vi "Plot_Server_Data.vi"() -> ()   [LabVIEW 2021]
uses:
  Anemometry/Anemometry Sub Vis/Controls/Server_Comms.ctl
  Anemometry/Anemometry Sub Vis/File/Setup_Filetype.ctl
  Anemometry/Anemometry Sub Vis/Globals/Preference_global.vi
  ADAM Server/ADAM_Global.vi
panel:
  out "LastUpdated":string="Tue, May 12, 2015 at 11:28"
  in  "Throwback\n(mins)":dbl format="%.1f"
  in  "stop":bool=TRUE
  in  "Mode":T1(ring)=enum."Display data over specified period:"
  in  "History\n(mins)":dbl=20.0 format="%.1f"
  in  "Save plot number":T2(ring)
  out "Plot 3 Chs":string[](array[string])
  out "Plot 2 Chs":string[](array[string])
  out "Plot 1 Chs":string[](array[string])
  in  "Selector 1":i32[](listbox)
  in  "Search 1":string caption="Search:"
  in  "Search 2":string caption="Search:"
  in  "Search 3":string caption="Search:"
  in  "Selector 3":i32[](listbox)
  in  "Selector 2":i32[](listbox)
  in  "Precision":i32=2
  in  "Save 3":bool
  in  "palette3":i32(ring)=5 caption="Palette" items=["Strong", "Dark", "Light", "Pastel", "Pale", "Brash", "Clean", "Tidy"]
  out "Plot 3":cluster{"Times":dbl[], "Output array":dbl[]}[](graph)
  in  "Save 2":bool
  in  "palette2":i32(ring)=5 caption="Palette" items=["Strong", "Dark", "Light", "Pastel", "Pale", "Brash", "Clean", "Tidy"]
  out "Plot 2":cluster{"Times":dbl[], "Output array":dbl[]}[](graph)
  in  "Save 1":bool
  in  "palette1":i32(ring)=5 caption="Palette" items=["Strong", "Dark", "Light", "Pastel", "Pale", "Brash", "Clean", "Tidy"]
  out "Plot 1":cluster{"Times":dbl[], "Output array":dbl[]}[](graph)
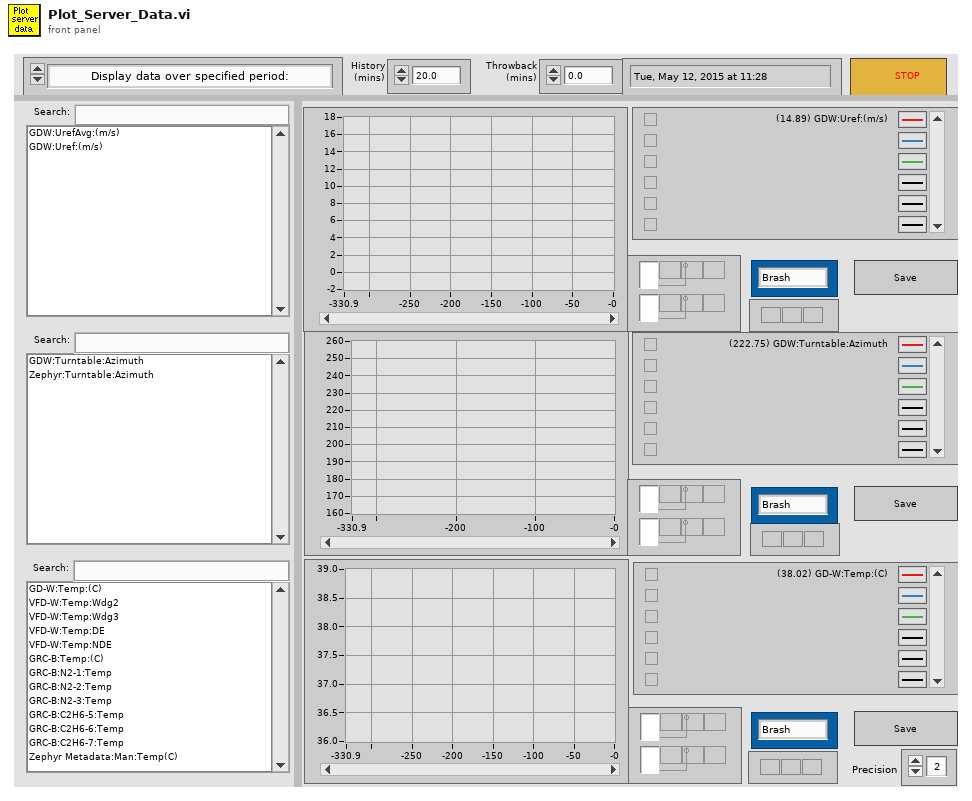
[diagram p1: front panel]
types:
  T1 = enum16{"Display full time history", "Display data over specified period:"}
  T2 = enum16{"Save Plot 1", "Save Plot 2", "Save Plot 3"}
  T3 = typedef "Server_Comms.ctl" = enum16{"Do Not Link To Server", "Server Link Healthy"}
  T4 = typedef "Setup_Filetype.ctl" = enum16{"Measurement Setups", "Calibration Setups", "General", "Results File Plotter Setups", "Speed Calib Tweaks"}
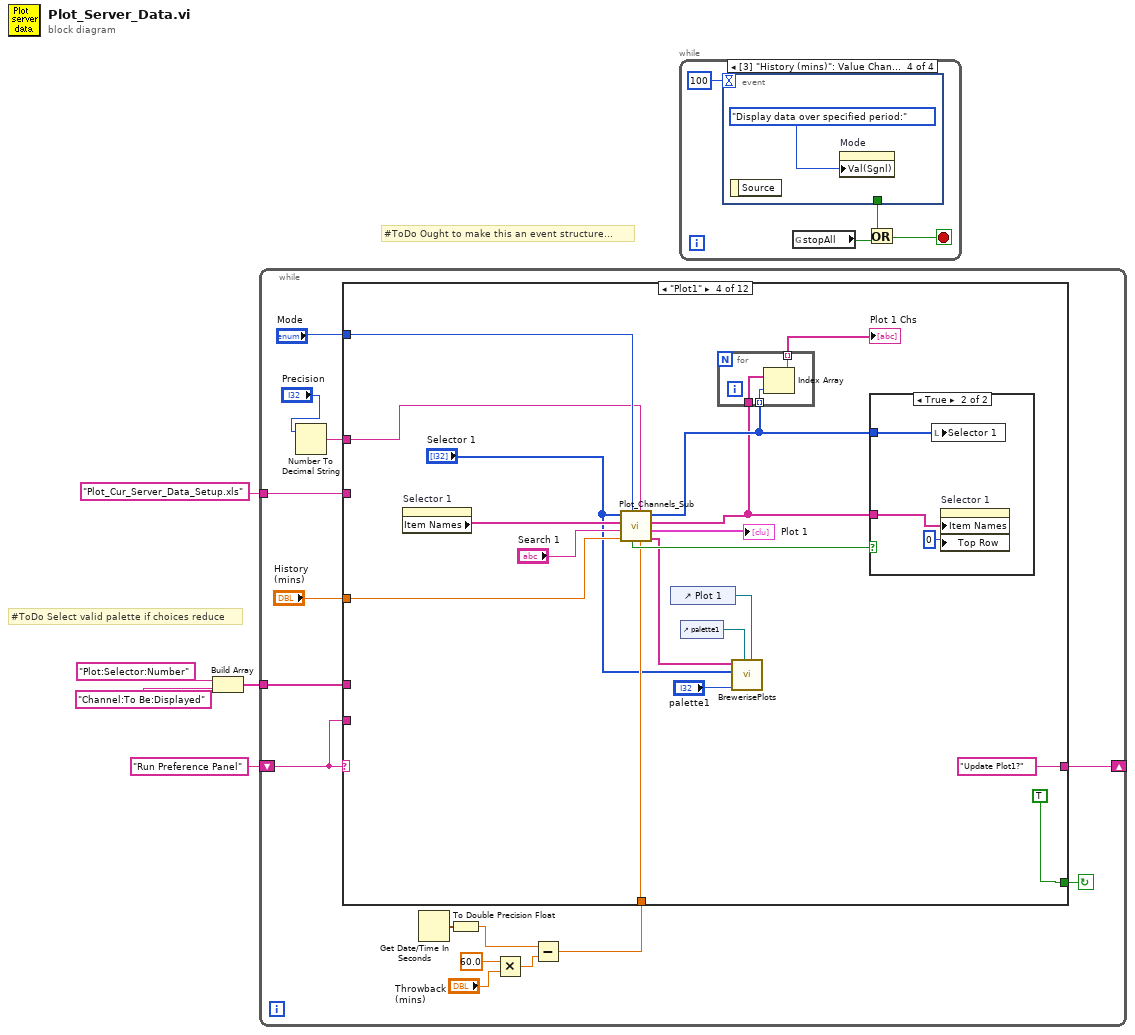
[diagram p0: block diagram]
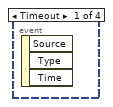
[diagram p2: hidden frame]
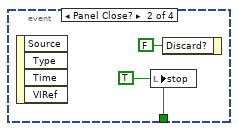
[diagram p3: hidden frame]
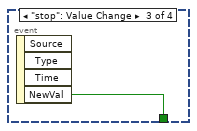
[diagram p4: hidden frame]
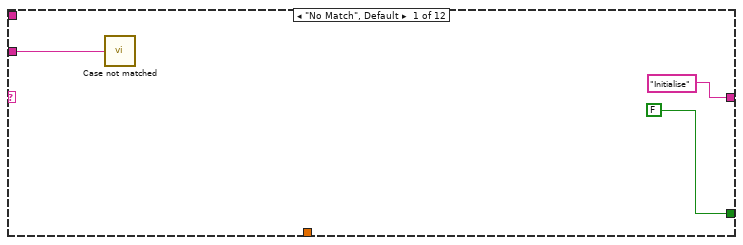
[diagram p5: hidden frame]
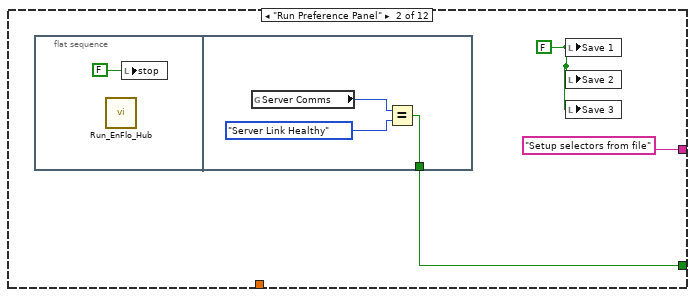
[diagram p6: hidden frame]
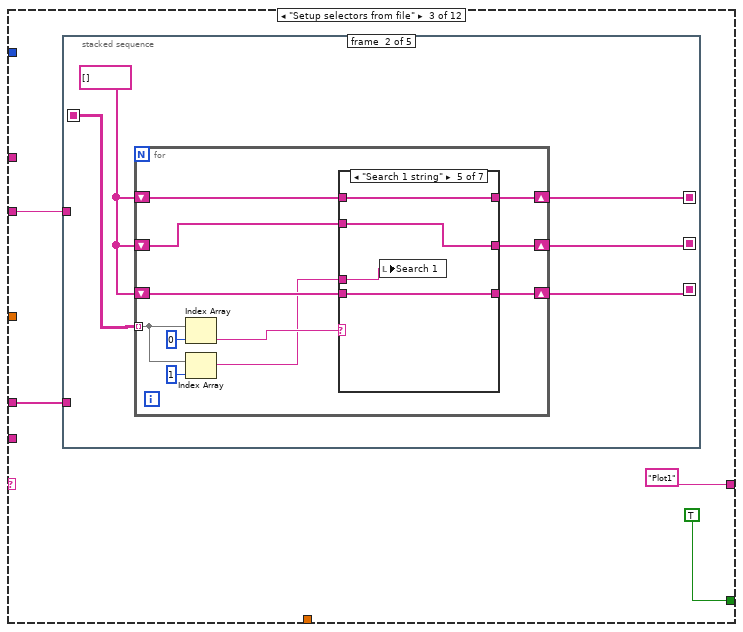
[diagram p7: hidden frame]
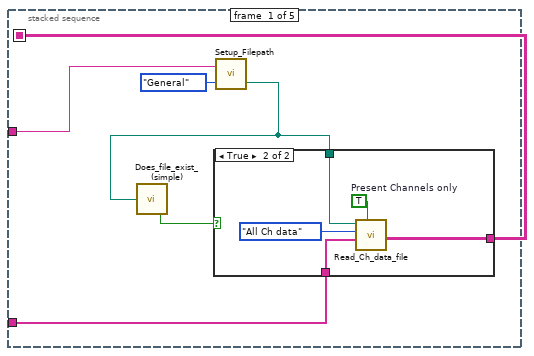
[diagram p8: hidden frame]
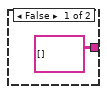
[diagram p9: hidden frame]
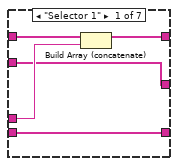
[diagram p10: hidden frame]
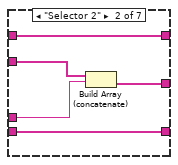
[diagram p11: hidden frame]
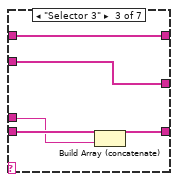
[diagram p12: hidden frame]
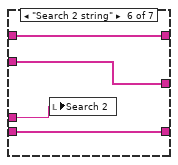
[diagram p14: hidden frame]
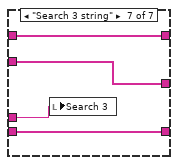
[diagram p15: hidden frame]
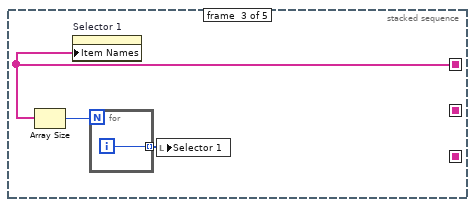
[diagram p16: hidden frame]
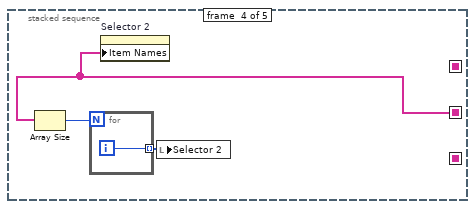
[diagram p17: hidden frame]
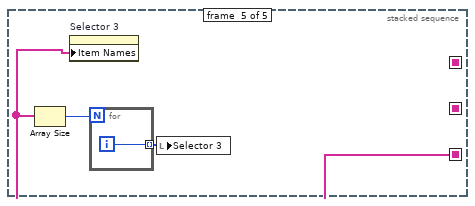
[diagram p18: hidden frame]
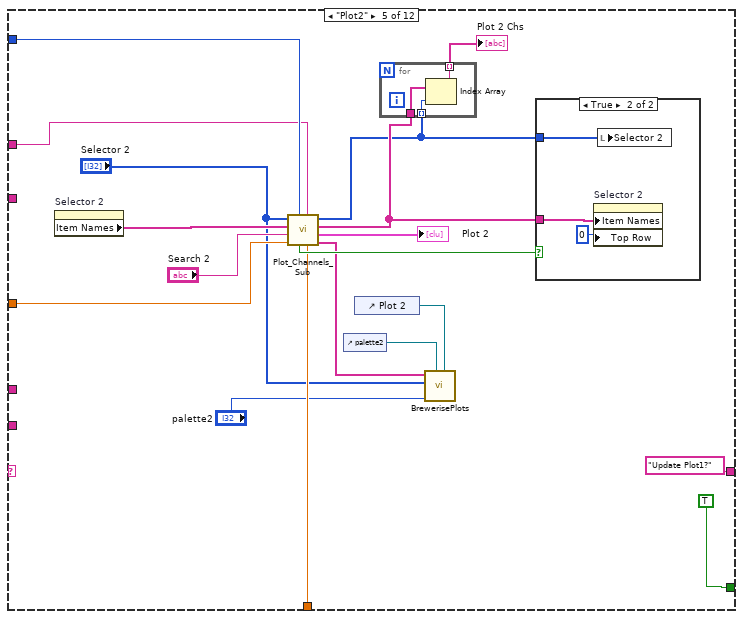
[diagram p20: hidden frame]
diagram:
  # "#ToDo Select valid palette if choices reduce"
  # "#ToDo Ought to make this an event structure..."
  n1 = Build Array("Plot:Selector:Number", "Channel:To Be:Displayed") -> (w2:string[])
  n2 = while {
    shift-left: "Run Preference Panel" -> [w18]
    shift-right: [w19] -> _
    tunnel: w2 -> [w15]
    tunnel: "Plot_Cur_Server_Data_Setup.xls" -> [w14]
    stop <- w20 continue-if-true
    n3 = Number To Decimal String(number="Precision") -> (decimal integer string=w12:string)  [unwired: 1 out]
    n4 = Get Date/Time In Seconds() -> (seconds since 1Jan1904=w11:timestamp)
    n5 = To Double Precision Float(number=w11) -> (double precision float=w7:dbl)
    n6 = Multiply(x=60.0, y="Throwback\n(mins)") -> (x*y=w8:dbl)
    n7 = Subtract(x=w7, y=w8) -> (x-y=w6:dbl)
    n8 = case shown="\"Plot1\"" w18 {
      tunnel: [FALSE w25 TRUE TRUE TRUE TRUE TRUE TRUE TRUE TRUE w319 w385] -> w20
      tunnel: ["Initialise" "Setup selectors from file" "Plot1" "Update Plot1?" "Update Plot1?" "Update Plot1?" w181 w207 w232 w267 w320 "Update Plot1?" ("t")] -> w19
      tunnel: w18 -> [w21 _ _ _ _ _ _ _ _ _ _ _]
      tunnel: "Mode" -> [_ _ _ w116 w143 w167 _ _ _ _ _ _]
      tunnel: "History\n(mins)" -> [_ _ _ w115 w142 w166 _ _ _ _ _ _]
      tunnel: w15 -> [_ _ w31 _ _ _ _ _ _ _ _ w389]
      tunnel: w14 -> [_ _ w32 _ _ _ _ _ _ _ _ w388]
      tunnel: w12 -> [_ _ _ w111 w135 w159 _ _ _ _ _ _]
      tunnel: w6 -> [_ _ _ w110 w134 w158 _ _ _ _ _ _]
      frame "No Match", Default {
        n9 = call "Case not matched.vi"("Case Name not Matched"=w21) -> ()
      }
      frame "Run Preference Panel" {
        w24 = FALSE ("Save 1")
        n10 = flat-sequence {
          tunnel: [w28] -> w25
          frame #0 {
            n11 = call "Run_EnFlo_Hub.vi"() -> ()  [unwired: 1 in, 7 out]
            n12 = local write "stop"(FALSE ("stop")) -> ()
          }
          frame #1 {
            n13 = global read "Preference_global.vi" "Server Comms"() -> (w29:T3)
            n14 = Equal?(x=w29, y=Server_Comms."Server Link Healthy" ("Server Comms")) -> (x = y?=w28:bool)
          }
        }
        n15 = local write "Save 1"(w24) -> ()
        n16 = local write "Save 2"(w24) -> ()
        n17 = local write "Save 3"(w24) -> ()
      }
      frame "Setup selectors from file" {
        n18 = stacked-sequence {
          seq-local: [w38 _ _ _ _] -> [_ w51 _ _ _]
          seq-local: [_ w49 _ _ _] -> [_ _ w95 _ _]
          seq-local: [_ w47 _ _ _] -> [_ _ _ w97 _]
          seq-local: [_ w48 _ _ _] -> [_ _ _ _ w101]
          tunnel: w32 -> [w37 _ _ _ _]
          tunnel: w31 -> [w39 _ _ _ _]
          frame #0 {
            n19 = call "Setup_Filepath.vi"("Setup File Type"=Setup_Filetype."General", "Filename in"=w37) -> ("Filename Out"=w36:path)  [unwired: 1 out]
            n20 = call "Does_file_exist_(simple).vi"("Pathname"=w36) -> ("exists?"=w40:bool)
            n21 = case shown="True" w40 {
              tunnel: w36 -> [_ w46]
              tunnel: w39 -> [_ w45]
              tunnel: [string[][] [] ("Channel Values") w42] -> w38
              frame False {
              }
              frame True {
                w44 = TRUE  # Present Channels only
                n22 = call "Read_Ch_data_file.vi"("Present Channels only"=w44, "Present Channels"=w45, "Output"=enum16{"All Ch data", "The last few rows"}."All Ch data", "Filename"=w46) -> ("Channel Values"=w42:string[][])  [unwired: 1 in, 4 out]
              }
            }
          }
          frame #1 {
            w50 = string[] []
            n23 = for {
              shift-right: [w57] -> w49
              shift-left: w50 -> [w58]
              tunnel: w51 -> [w59] mode=indexing
              shift-right: [w55] -> w47
              shift-left: w50 -> [w56]
              shift-right: [w53] -> w48
              shift-left: w50 -> [w54]
              n24 = Index Array(array=w59, index=0 ("Index")) -> (element=w61:string)
              n25 = Index Array(array=w59, index=1 ("Index")) -> (element=w52:string)
              n26 = case shown="\"Search 1 string\"" w61 {
                tunnel: w58 -> [w67 w72 w73 w79 w83 w87 w91]
                tunnel: [w66 w72 w73 w79 w83 w87 w91] -> w57
                tunnel: w52 -> [w65 w69 w75 _ w81 w85 w89]
                tunnel: w56 -> [w64 w70 w74 w80 w84 w88 w92]
                tunnel: [w64 w68 w74 w80 w84 w88 w92] -> w55
                tunnel: w54 -> [w63 w71 w77 w78 w82 w86 w90]
                tunnel: [w63 w71 w76 w78 w82 w86 w90] -> w53
                frame "Selector 1" {
                  n27 = Build Array (concatenate)(w67, w65) -> (w66:string[])
                }
                frame "Selector 2" {
                  n28 = Build Array (concatenate)(w70, w69) -> (w68:string[])
                }
                frame "Selector 3" {
                  n29 = Build Array (concatenate)(w77, w75) -> (w76:string[])
                }
                frame "No Match", Default {
                }
                frame "Search 1 string" {
                  n30 = local write "Search 1"(w81) -> ()
                }
                frame "Search 2 string" {
                  n31 = local write "Search 2"(w85) -> ()
                }
                frame "Search 3 string" {
                  n32 = local write "Search 3"(w89) -> ()
                }
              }
            }
          }
          frame #2 {
            n33 = Array Size(array=w95) -> (size(s)=w94:i32)
            n34 = property on="Selector 1" class="LstBox (strict)"("Item Names"=w95) -> ()  [unwired: 2 in, 2 out]
            n35 = for {
              N: w94 -> [_]
              tunnel: [w96] -> w93 mode=indexing
              i -> [w96]
            }
            n36 = local write "Selector 1"(w93) -> ()
          }
          frame #3 {
            n37 = Array Size(array=w97) -> (size(s)=w99:i32)
            n38 = for {
              N: w99 -> [_]
              tunnel: [w100] -> w98 mode=indexing
              i -> [w100]
            }
            n39 = property on="Selector 2" class="LstBox (strict)"("Item Names"=w97) -> ()  [unwired: 2 in, 2 out]
            n40 = local write "Selector 2"(w98) -> ()
          }
          frame #4 {
            n41 = Array Size(array=w101) -> (size(s)=w103:i32)
            n42 = property on="Selector 3" class="LstBox (strict)"("Item Names"=w101) -> ()  [unwired: 2 in, 2 out]
            n43 = for {
              N: w103 -> [_]
              tunnel: [w104] -> w102 mode=indexing
              i -> [w104]
            }
            n44 = local write "Selector 3"(w102) -> ()
          }
        }
      }
      frame "Plot1" {
        n45 = property on="Selector 1" class="LstBox (strict)"() -> ("Item Names"=w117:string[])  [unwired: 2 in, 2 out]
        n46 = call "Plot_Channels_Sub.vi"("End Time"=w110, "precision"=w111, "Mode"=w116, "History (min)"=w115, "Search String"="Search 1", "Selector List In"=w117, "Selector array In"="Selector 1") -> ("Plot Legend"=w107:string[], "Plot"=→"Plot 1":cluster{"Times":dbl[], "Output array":dbl[]}[], "Selector List Out"=w113:string[], "Selector array Out"=w114:i32[], "Selector Changed?"=w119:bool)
        n47 = control-ref of="Plot 1"() -> (w109:refnum<vi>)
        n48 = control-ref of="palette1"() -> (w108:refnum<vi>)
        n49 = for {
          tunnel: w114 -> [w125] mode=indexing
          tunnel: w113 -> [w124]
          tunnel: [w123] -> w112 mode=indexing
          n50 = Index Array(array=w124, index=w125) -> (element=w123:string)
        }
        "Plot 1 Chs" <- w112
        n51 = call "BrewerisePlots.vi"("graphRefnum"=w109, "paletteRefnum"=w108, "paletteNum"="palette1", "Series"="Selector 1", "Plot Legends"=w107) -> ()  [unwired: 7 in]
        n52 = case shown="True" w119 {
          tunnel: w113 -> [_ w128]
          tunnel: w114 -> [_ w127]
          frame False {
          }
          frame True {
            n53 = local write "Selector 1"(w127) -> ()
            n54 = property on="Selector 1" class="LstBox (strict)"("Item Names"=w128, "Top Row"=0) -> ()  [unwired: 2 in, 2 out]
          }
        }
      }
      frame "Plot2" {
        n55 = property on="Selector 2" class="LstBox (strict)"() -> ("Item Names"=w139:string[])  [unwired: 2 in, 2 out]
        n56 = call "Plot_Channels_Sub.vi"("End Time"=w134, "precision"=w135, "Mode"=w143, "History (min)"=w142, "Search String"="Search 2", "Selector List In"=w139, "Selector array In"="Selector 2") -> ("Plot Legend"=w131:string[], "Plot"=→"Plot 2":cluster{"Times":dbl[], "Output array":dbl[]}[], "Selector List Out"=w138:string[], "Selector array Out"=w137:i32[], "Selector Changed?"=w144:bool)
        n57 = control-ref of="palette2"() -> (w132:refnum<vi>)
        n58 = control-ref of="Plot 2"() -> (w133:refnum<vi>)
        n59 = for {
          tunnel: w137 -> [w149] mode=indexing
          tunnel: w138 -> [w148]
          tunnel: [w147] -> w136 mode=indexing
          n60 = Index Array(array=w148, index=w149) -> (element=w147:string)
        }
        "Plot 2 Chs" <- w136
        n61 = call "BrewerisePlots.vi"("graphRefnum"=w133, "paletteRefnum"=w132, "paletteNum"="palette2", "Series"="Selector 2", "Plot Legends"=w131) -> ()  [unwired: 7 in]
        n62 = case shown="True" w144 {
          tunnel: w138 -> [_ w151]
          tunnel: w137 -> [_ w152]
          frame False {
          }
          frame True {
            n63 = property on="Selector 2" class="LstBox (strict)"("Item Names"=w151, "Top Row"=0) -> ()  [unwired: 2 in, 2 out]
            n64 = local write "Selector 2"(w152) -> ()
          }
        }
      }
      frame "Plot3" {
        n65 = property on="Selector 3" class="LstBox (strict)"() -> ("Item Names"=w163:string[])  [unwired: 2 in, 2 out]
        n66 = call "Plot_Channels_Sub.vi"("End Time"=w158, "precision"=w159, "Mode"=w167, "History (min)"=w166, "Search String"="Search 3", "Selector List In"=w163, "Selector array In"="Selector 3") -> ("Plot Legend"=w155:string[], "Plot"=→"Plot 3":cluster{"Times":dbl[], "Output array":dbl[]}[], "Selector List Out"=w162:string[], "Selector array Out"=w161:i32[], "Selector Changed?"=w168:bool)
        n67 = control-ref of="Plot 3"() -> (w157:refnum<vi>)
        n68 = control-ref of="palette3"() -> (w156:refnum<vi>)
        n69 = for {
          tunnel: w161 -> [w173] mode=indexing
          tunnel: w162 -> [w172]
          tunnel: [w171] -> w160 mode=indexing
          n70 = Index Array(array=w172, index=w173) -> (element=w171:string)
        }
        "Plot 3 Chs" <- w160
        n71 = call "BrewerisePlots.vi"("graphRefnum"=w157, "paletteRefnum"=w156, "paletteNum"="palette3", "Series"="Selector 3", "Plot Legends"=w155) -> ()  [unwired: 7 in]
        n72 = case shown="True" w168 {
          tunnel: w162 -> [_ w175]
          tunnel: w161 -> [_ w176]
          frame False {
          }
          frame True {
            n73 = local write "Selector 3"(w176) -> ()
            n74 = property on="Selector 3" class="LstBox (strict)"("Item Names"=w175, "Top Row"=0) -> ()  [unwired: 2 in, 2 out]
          }
        }
      }
      frame "Update Plot1?" {
        n75 = while {
          shift-right: [w201] -> w188
          shift-left: _ -> [w198]
          shift-right: [w200] -> w190
          shift-left: _ -> [w199]
          tunnel: [w199] -> w189
          tunnel: [w198] -> w187
          shift-right: [w196] -> w178
          shift-left: _ -> [w195]
          tunnel: [w195] -> w179
          stop <- FALSE continue-if-true
          n76 = local read "Selector 1"() -> (w201:i32[])
          n77 = local read "palette1"() -> (w196:i32)
          n78 = local read "Search 1"() -> (w200:string)
        }
        n79 = case shown="False" "Save 1" {
          tunnel: ["Update Plot2?" "Save Plot" ("t")] -> w180
          frame False {
          }
          frame True {
            n80 = local write "Save plot number"(T2."Save Plot 1" ("Save plot number")) -> ()
          }
        }
        n81 = Equal?(x=w178, y=w179) -> (x = y?=w177:bool)
        n82 = Equal?(x=w188, y=w187) -> (x = y?=w185:bool)
        n83 = Equal?(x=w189, y=w190) -> (x = y?=w186:bool)
        n84 = Compound Arithmetic op=AND(w177, w185, w186) -> (w184:bool)
        n85 = Select(t=w180, s=w184, f="Plot1") -> (s? t:f=w181:string)
      }
      frame "Update Plot2?" {
        n86 = while {
          shift-right: [w226] -> w213
          shift-left: _ -> [w223]
          shift-right: [w225] -> w215
          shift-left: _ -> [w224]
          tunnel: [w224] -> w214
          tunnel: [w223] -> w212
          shift-right: [w221] -> w203
          shift-left: _ -> [w220]
          tunnel: [w220] -> w204
          stop <- FALSE continue-if-true
          n87 = local read "Selector 2"() -> (w226:i32[])
          n88 = local read "Search 2"() -> (w225:string)
          n89 = local read "palette2"() -> (w221:i32)
        }
        n90 = case shown="False" "Save 2" {
          tunnel: ["Update Plot3?" "Save Plot" ("t")] -> w205
          frame False {
          }
          frame True {
            n91 = local write "Save plot number"(T2."Save Plot 2" ("Save plot number")) -> ()
          }
        }
        n92 = Equal?(x=w203, y=w204) -> (x = y?=w202:bool)
        n93 = Equal?(x=w213, y=w212) -> (x = y?=w210:bool)
        n94 = Equal?(x=w214, y=w215) -> (x = y?=w211:bool)
        n95 = Compound Arithmetic op=AND(w202, w210, w211) -> (w209:bool)
        n96 = Select(t=w205, s=w209, f="Plot2") -> (s? t:f=w207:string)
      }
      frame "Update Plot3?" {
        n97 = while {
          shift-right: [w251] -> w238
          shift-left: _ -> [w248]
          shift-right: [w250] -> w240
          shift-left: _ -> [w249]
          tunnel: [w249] -> w239
          tunnel: [w248] -> w237
          shift-right: [w246] -> w229
          shift-left: _ -> [w245]
          tunnel: [w245] -> w228
          stop <- FALSE continue-if-true
          n98 = local read "Selector 3"() -> (w251:i32[])
          n99 = local read "Search 3"() -> (w250:string)
          n100 = local read "palette3"() -> (w246:i32)
        }
        n101 = case shown="False" "Save 3" {
          tunnel: ["What to do next?" "Save Plot" ("t")] -> w230
          frame False {
          }
          frame True {
            n102 = local write "Save plot number"(T2."Save Plot 3" ("Save plot number")) -> ()
          }
        }
        n103 = Equal?(x=w238, y=w237) -> (x = y?=w235:bool)
        n104 = Equal?(x=w239, y=w240) -> (x = y?=w236:bool)
        n105 = Equal?(x=w229, y=w228) -> (x = y?=w227:bool)
        n106 = Compound Arithmetic op=AND(w227, w235, w236) -> (w234:bool)
        n107 = Select(t=w230, s=w234, f="Plot3") -> (s? t:f=w232:string)
      }
      frame "What to do next?" {
        n108 = Wait (ms)(milliseconds to wait=u32 300) -> ()  [unwired: 1 out]
        n109 = while {
          shift-right: [w283] -> _
          shift-left: _ -> [w282]
          shift-right: [w281] -> _
          shift-left: _ -> [w280]
          shift-right: [w273] -> _
          shift-left: _ -> [w272]
          tunnel: [w275] -> w266
          shift-right: [w269] -> w256
          shift-left: _ -> [w270]
          stop <- FALSE continue-if-true
          n110 = local read "History\n(mins)"() -> (w283:dbl)
          n111 = local read "Mode"() -> (w281:T1)
          n112 = Equal?(x=w283, y=w282) -> (x = y?=w279:bool)
          n113 = Equal?(x=w280, y=w281) -> (x = y?=w278:bool)
          n114 = And(x=w279, y=w278) -> (x .and. y?=w277:bool)
          n115 = Select(t=w272, s=w277, f=0) -> (s? t:f=w274:i32)
          n116 = case shown="5" w274 {
            tunnel: ["Plot1" "Plot2" "Plot3" "Update Plot1?" "Update Plot1?" "Update Plot1?" "Update Plot1?"] -> w275
            tunnel: w274 -> [w286 w290 w294 w300 w306 w312 _]
            tunnel: [w285 w289 w293 w299 w305 w311 0] -> w273
            tunnel: w270 -> [w284 w288 w292 w297 w303 w308 w315]
            tunnel: [w284 w288 w292 w296 w302 w309 w314] -> w269
            frame 0, Default {
              n117 = Increment(x=w286) -> (x+1=w285:i32)
            }
            frame 1 {
              n118 = Increment(x=w290) -> (x+1=w289:i32)
            }
            frame 2 {
              n119 = Increment(x=w294) -> (x+1=w293:i32)
            }
            frame 3 {
              n120 = Add(x=w297, y=1) -> (x+y=w296:i32)
              n121 = Increment(x=w300) -> (x+1=w299:i32)
            }
            frame 4 {
              n122 = Add(x=w303, y=1) -> (x+y=w302:i32)
              n123 = Increment(x=w306) -> (x+1=w305:i32)
            }
            frame 5 {
              n124 = Add(x=w308, y=1) -> (x+y=w309:i32)
              n125 = Increment(x=w312) -> (x+1=w311:i32)
            }
            frame 6 {
              n126 = Add(x=w315, y=1) -> (x+y=w314:i32)
            }
          }
        }
        n127 = Get Date/Time String(date format (0)=enum16{"short", "long", "abbreviated"}."abbreviated") -> (date string=w263:string, time string=w264:string)  [unwired: 2 out]
        n128 = Concatenate Strings(w263, " at " ("Substring"), w264) -> (→"LastUpdated":string)
        n129 = Quotient & Remainder(x=w256, y=500) -> (x-y*floor(x/y)=w260:i32)  [unwired: 1 out]
        n130 = global read "ADAM_Global.vi" "stopAll"() -> (w252:bool)
        n131 = Equal To 0?(x=w260) -> (x = 0?=w258:bool)
        n132 = Compound Arithmetic op=OR("stop", w258, w252) -> (w257:bool)
        n133 = Select(t="Save Channel Names", s=w257, f=w266) -> (s? t:f=w267:string)
      }
      frame "Save Plot" {
        n134 = stacked-sequence {
          seq-local: [w331 _] -> [_ w359]
          seq-local: [w326 _] -> [_ w361]
          seq-local: [w330 _] -> [_ w360]
          seq-local: [w321 _] -> [_ w349]
          tunnel: ["What to do next?" _] -> w320
          tunnel: [TRUE _] -> w319
          frame #0 {
            n135 = case shown="\"Save Plot 1\"" "Save plot number" {
              tunnel: [w339 w342 w345] -> w336
              tunnel: [w338 w341 w344] -> w331
              frame "Save Plot 1" {
                n136 = local read "Plot 1 Chs"() -> (w338:string[])
                n137 = local write "Save 1"(FALSE ("Save 1")) -> ()
                n138 = local read "Plot 1"() -> (w339:cluster{"Times":dbl[], "Output array":dbl[]}[])
              }
              frame "Save Plot 2" {
                n139 = local read "Plot 2 Chs"() -> (w341:string[])
                n140 = local write "Save 2"(FALSE ("Save 1")) -> ()
                n141 = local read "Plot 2"() -> (w342:cluster{"Times":dbl[], "Output array":dbl[]}[])
              }
              frame "Save Plot 3" {
                n142 = local read "Plot 3 Chs"() -> (w344:string[])
                n143 = local write "Save 3"(FALSE ("Save 1")) -> ()
                n144 = local read "Plot 3"() -> (w345:cluster{"Times":dbl[], "Output array":dbl[]}[])
              }
            }
            n145 = Index Array(array=w336, index=0) -> (element=w334:cluster{"Times":dbl[], "Output array":dbl[]})
            n146 = Unbundle(w334) -> ("Times"=w325:dbl[])  [unwired: 1 out]
            n147 = Get Date/Time In Seconds() -> (seconds since 1Jan1904=w328:timestamp)
            n148 = for {
              tunnel: w336 -> [w347] mode=indexing
              tunnel: [w346] -> w330 mode=indexing
              n149 = Unbundle(w347) -> ("Output array"=w346:dbl[])  [unwired: 1 out]
            }
            n150 = To Double Precision Float(number=w328) -> (double precision float=w327:dbl)
            n151 = Multiply(x=w325, y=60.0) -> (x*y=w323:dbl[])
            n152 = Add(x=w327, y=w323) -> (x+y=w326:dbl[])
            n153 = Index Array(array=w323) -> (element=w322:dbl)  [unwired: 1 in]
            n154 = Subtract(x=w323, y=w322) -> (x-y=w321:dbl[])
          }
          frame #1 {
            w354 = FALSE  # append to file? (new file:F)
            n155 = for {
              tunnel: w360 -> [w381]
              tunnel: w361 -> [w375] mode=indexing
              tunnel: [w377] -> w353 mode=indexing
              tunnel: w349 -> [w371] mode=indexing
              i -> [w380]
              n156 = Number To Decimal String(number=w375) -> (decimal integer string=w376:string)  [unwired: 1 out]
              n157 = Index Array(array=w381, index (col)=w380) -> (element=w379:dbl[])  [unwired: 1 in]
              n158 = Number To Fractional String(number=w371, precision (6)=i16 2) -> (F-format string=w370:string)  [unwired: 2 in]
              n159 = Get Date/Time String(seconds (now)=w375) -> (date string=w374:string, time string=w373:string)  [unwired: 2 out]
              n160 = for {
                tunnel: w379 -> [w383] mode=indexing
                tunnel: [w382] -> w378 mode=indexing
                n161 = call "Number_2_string.vi"("number"=w383) -> ("String"=w382:string)  [unwired: 1 in]
              }
              n162 = Build Array (concatenate)(w374, w373, w376, w370, w378) -> (w377:string[])
            }
            n163 = Build Array (concatenate)("Date::", "Centre:Time:", "Seconds:Since:1st Jan 1904", "Time:in:Seconds", w359) -> (w352:string[])
            n164 = call "Ch_names_to_rows.vi"("Channel Names"=w352) -> ("3 Row names"=w358:string[][])
            n165 = File Dialog(7:"Please choose file name" ("prompt")) -> (3:w366:path)  [unwired: 1 in, 8 out]
            n166 = Build Array (concatenate)(w358, w353) -> (w356:string[][])
            n167 = Strip Path(path=w366) -> (stripped path=w363:path, name=w365:string)
            n168 = call "Add_filename_suffix.vi"("Filename"=w365, "Suffix to add"=".xls") -> ("Filename out"=w362:string)  [unwired: 3 out]
            n169 = Array To Spreadsheet String(array=w356, 3:"%s" ("format string")) -> (spreadsheet string=w355:string)  [unwired: 1 out]
            n170 = Build Path(base path=w363, name or relative path=w362) -> (appended path=w351:path)
            n171 = call "Write_File_Simple.vi"("append to file? (new file:F)"=w354, "character string"=w355, "file path"=w351) -> ()  [unwired: 2 out]
          }
        }
      }
      frame "Save Channel Names" {
        n172 = stacked-sequence {
          seq-local: [w391 _ _] -> [_ w415 _]
          seq-local: [_ w414 _] -> [_ _ w428]
          tunnel: w389 -> [_ _ w429]
          tunnel: w388 -> [_ _ w426]
          frame #0 {
            n173 = for {
              N: 3 -> [_]
              shift-right: [w395] -> w391
              shift-left: string[][] [] -> [w397]
              i -> [w402]
              n174 = Increment(x=w402) -> (x+1=w399:i32)
              n175 = case shown="1, Default" w399 {
                tunnel: [w409 w410 w412] -> w401
                tunnel: [w408 w411 w413] -> w393
                frame 1, Default {
                  n176 = local read "Selector 1"() -> (w409:i32[])
                  n177 = property on="Selector 1" class="LstBox (strict)"() -> ("Item Names"=w408:string[])  [unwired: 2 in, 2 out]
                }
                frame 2 {
                  n178 = property on="Selector 2" class="LstBox (strict)"() -> ("Item Names"=w411:string[])  [unwired: 2 in, 2 out]
                  n179 = local read "Selector 2"() -> (w410:i32[])
                }
                frame 3 {
                  n180 = local read "Selector 3"() -> (w412:i32[])
                  n181 = property on="Selector 3" class="LstBox (strict)"() -> ("Item Names"=w413:string[])  [unwired: 2 in, 2 out]
                }
              }
              n182 = Format Into String(format string="%d" ("Format String"), initial string="Selector ", w399) -> (resulting string=w396:string)  [unwired: 1 in, 1 out]
              n183 = for {
                tunnel: w401 -> [w407] mode=indexing
                tunnel: w396 -> [w406]
                tunnel: [w404] -> w394 mode=indexing
                tunnel: w393 -> [w403]
                n184 = Index Array(array=w403, index=w407) -> (element=w405:string)
                n185 = Build Array(w406, w405) -> (w404:string[])
              }
              n186 = Build Array (concatenate)(w397, w394) -> (w395:string[][])
            }
          }
          frame #1 {
            n187 = local read "Search 1"() -> (w416:string)
            n188 = local read "Search 2"() -> (w417:string)
            n189 = local read "Search 3"() -> (w418:string)
            n190 = Build Array("Search 1 string" ("element"), w416) -> (w422:string[])
            n191 = Build Array("Search 3 string" ("element"), w418) -> (w424:string[])
            n192 = Build Array("Search 2 string" ("element"), w417) -> (w423:string[])
            n193 = Build Array (concatenate)(w415, w422, w423, w424) -> (w414:string[][])
          }
          frame #2 {
            n194 = call "Setup_Filepath.vi"("Setup File Type"=Setup_Filetype."General", "Filename in"=w426) -> ("Filename Out"=w425:path)  [unwired: 1 out]
            n195 = Array Size(array=w428) -> (size(s)=w432:i32[])
            n196 = Index Array(array=w432, index=1 ("Index")) -> (element=w431:i32)
            n197 = Not Equal To 0?(x=w431) -> (x != 0?=w430:bool)
            n198 = case shown="True" w430 {
              tunnel: w425 -> [w434 w439]
              tunnel: w428 -> [_ w440]
              tunnel: w429 -> [_ w441]
              frame False {
                n199 = Delete(path (use dialog)=w434) -> ()  [unwired: 1 in, 6 out]
              }
              frame True {
                w435 = FALSE  # append to file? (new file:F)
                n200 = call "Ch_names_to_rows.vi"("Channel Names"=w441) -> ("3 Row names"=w442:string[][])
                n201 = Build Array (concatenate)(w442, w440) -> (w437:string[][])
                n202 = Array To Spreadsheet String(array=w437, 3:"%s" ("format string")) -> (spreadsheet string=w436:string)  [unwired: 1 out]
                n203 = call "Write_File_Simple.vi"("append to file? (new file:F)"=w435, "character string"=w436, "file path"=w439) -> ()  [unwired: 2 out]
              }
            }
          }
        }
        n204 = global read "ADAM_Global.vi" "stopAll"() -> (w386:bool)
        n205 = local read "stop"() -> (w384:bool)
        n206 = Not Or(1:w384, 2:w386) -> (0:w385:bool)
      }
    }
  }
  n207 = while {
    stop <- w445 stop-if-true
    n208 = event shown="[3] \"History (mins)\": Value Change" {
      selector: _ -> [_ _ _ _]
      dyn-events: _ -> [_ _ _ _]
      timeout: 100 -> [_ _ _ _]
      tunnel: [_ w448 w449 _] -> w446
      event Timeout {
        n209 = event-data() -> ()  [unwired: 1 in, 3 out]
      }
      event Panel Close? {
        w448 = TRUE
        n210 = event-data() -> ()  [unwired: 1 in, 4 out]
        n211 = local write "stop"(w448) -> ()
        n212 = event-data("Discard?"=FALSE) -> ()  [unwired: 1 in, 1 out]
      }
      event "stop": Value Change {
        n213 = event-data() -> ("NewVal"=w449:bool)  [unwired: 1 in, 3 out]
      }
      event "History\n(mins)": Value Change {
        n214 = event-data() -> ()  [unwired: 1 in, 1 out]
        n215 = property on="Mode" class="Enum (strict)"("Val(Sgnl)"=T1."Display data over specified period:" ("Value (Signaling)")) -> ()  [unwired: 2 in, 2 out]
      }
    }
    n216 = global read "ADAM_Global.vi" "stopAll"() -> (w444:bool)
    n217 = Or(x=w446, y=w444) -> (x .or. y?=w445:bool)
  }
